vi "Two-TryGuessingGame_Branyon.vi"() -> ()   [LabVIEW 2019]
uses:
  <vilib>/numeric/Random Number (Range) U64.vi
  <vilib>/numeric/sub_Random U32.vi
panel:
  in  "Enter Guess 2":bool
  in  "Guess 2":u64
  out "number":u64
  in  "Guess":u64
  in  "Enter Guess":bool
  out "Message":string
  # "Gavin Branyon\n3/24/2024\nTwo-Try Guessing Game"
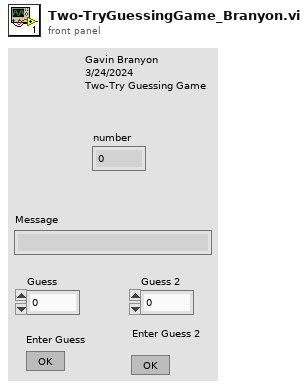
[diagram p1: front panel]
types:
  T1 = enum16{"Generate Number", "Guess", "Check Guess", "Check Guess 2", "Hint", "Correct", "Failure", "Guess 2"}
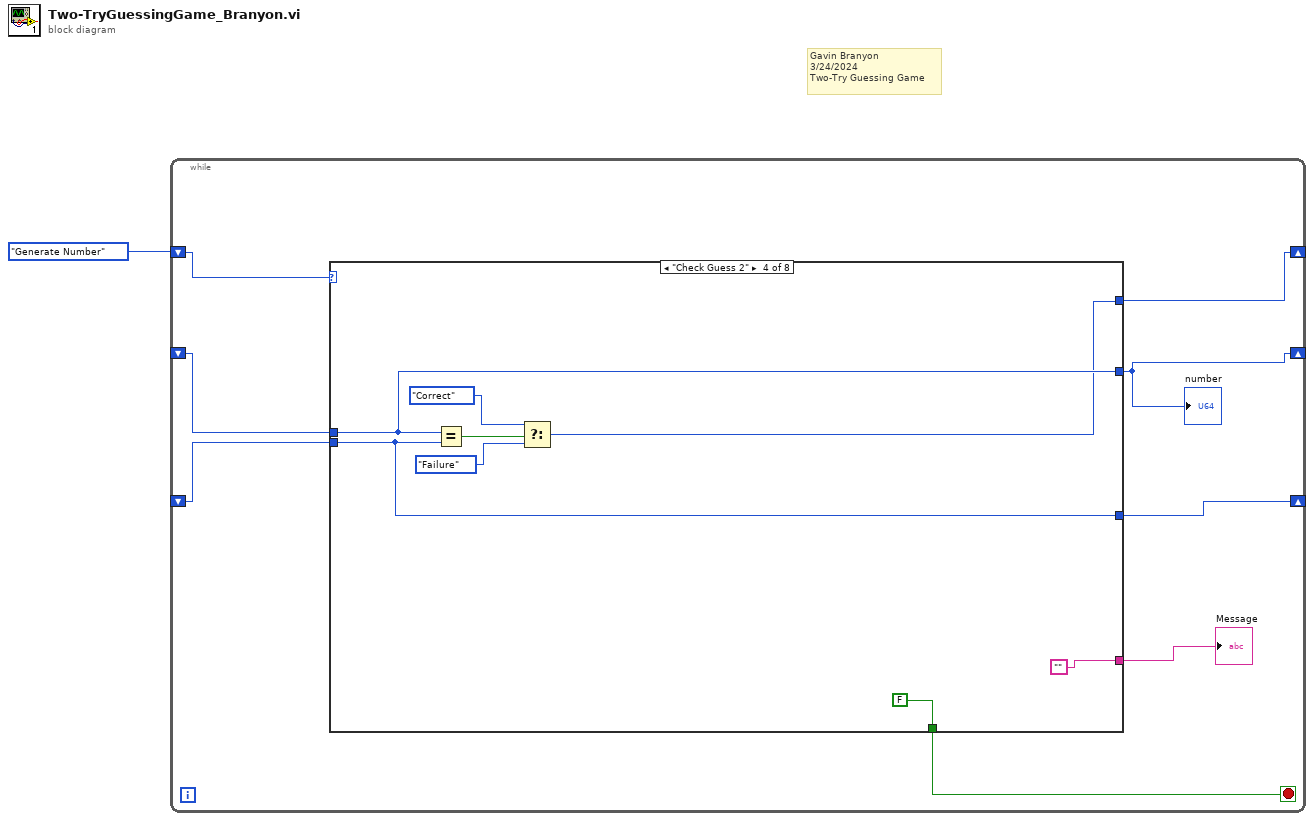
[diagram p0: block diagram]
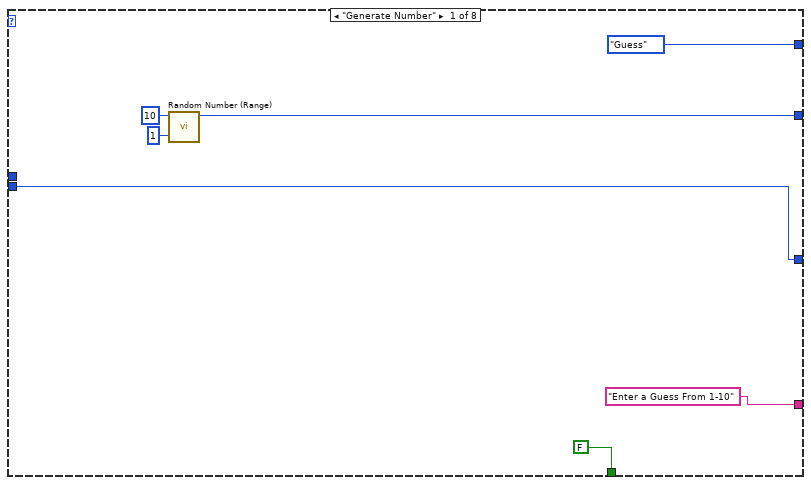
[diagram p2: hidden frame]
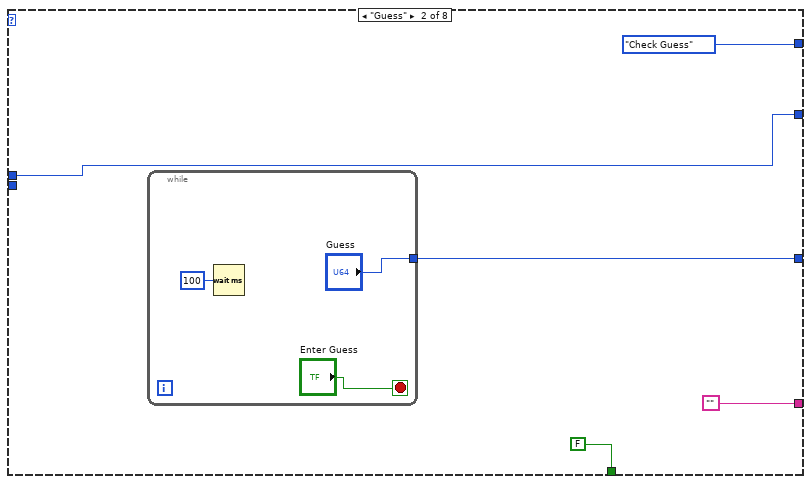
[diagram p3: hidden frame]
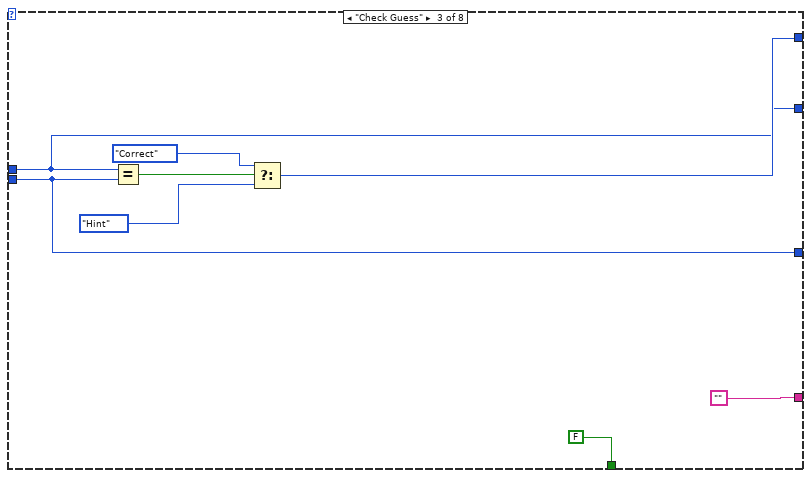
[diagram p4: hidden frame]
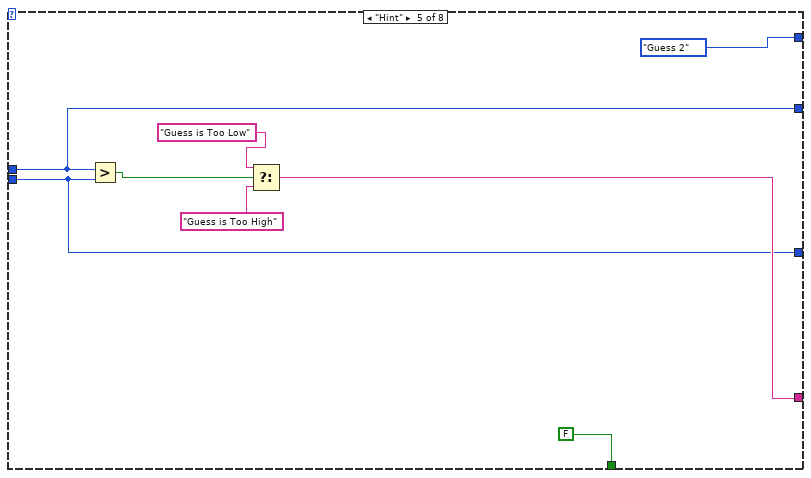
[diagram p5: hidden frame]
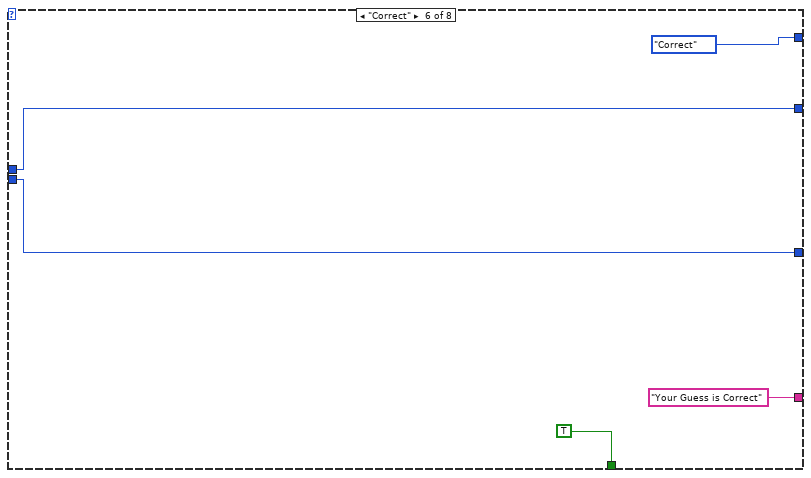
[diagram p6: hidden frame]
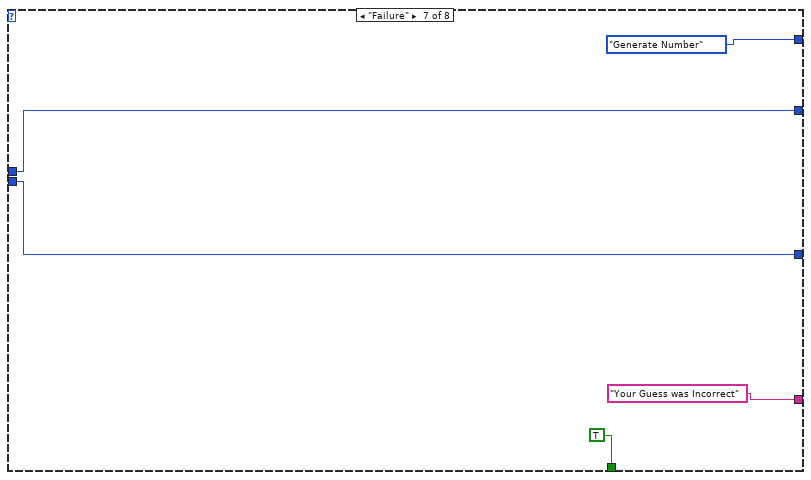
[diagram p7: hidden frame]
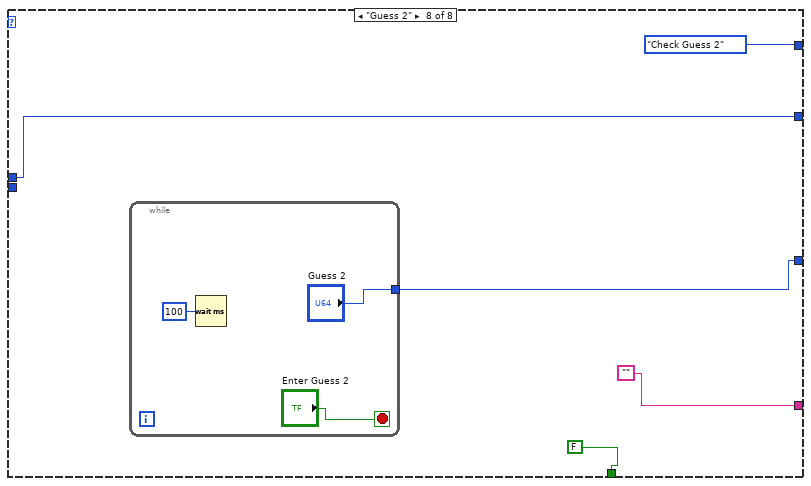
[diagram p8: hidden frame]
diagram:
  # "Gavin Branyon\n3/24/2024\nTwo-Try Guessing Game"
  n1 = while {
    shift-right: [w9] -> _
    shift-left: T1."Generate Number" -> [w3]
    shift-right: [w4] -> _
    shift-left: _ -> [w6]
    shift-right: [w7] -> _
    shift-left: _ -> [w5]
    stop <- w2 stop-if-true
    n2 = case shown="\"Check Guess 2\"" w3 {
      tunnel: [w14 w19 w30 w38 w43 w51 w58 w61] -> w4
      tunnel: [T1."Guess" T1."Check Guess" w31 w37 T1."Guess 2" T1."Correct" T1."Generate Number" T1."Check Guess 2"] -> w9
      tunnel: ["Enter a Guess From 1-10" "" "" "" w45 "Your Guess is Correct" "Your Guess was Incorrect" ""] -> w8
      tunnel: [w12 w21 w29 w39 w44 w52 w57 w62] -> w7
      tunnel: w6 -> [_ w19 w30 w38 w43 w51 w58 w61]
      tunnel: w5 -> [w12 _ w29 w39 w44 w52 w57 _]
      tunnel: [FALSE FALSE FALSE FALSE FALSE TRUE TRUE FALSE] -> w2
      frame "Generate Number" {
        n3 = call-poly <vilib>:"Random Number (Range).vi"("lower bound (0)"=u64 1, "upper bound (100)"=u64 10) -> ("number"=w14:u64)  [unwired: 9 in]
      }
      frame "Guess" {
        n4 = while {
          tunnel: ["Guess"] -> w21
          stop <- "Enter Guess" stop-if-true
          n5 = Wait (ms)(milliseconds to wait=u32 100) -> ()  [unwired: 1 out]
        }
      }
      frame "Check Guess" {
        n6 = Equal?(x=w30, y=w29) -> (x = y?=w32:bool)
        n7 = Select(t=T1."Correct", s=w32, f=T1."Hint") -> (s? t:f=w31:T1)
      }
      frame "Check Guess 2" {
        n8 = Equal?(x=w38, y=w39) -> (x = y?=w40:bool)
        n9 = Select(t=T1."Correct", s=w40, f=T1."Failure") -> (s? t:f=w37:T1)
      }
      frame "Hint" {
        n10 = Greater?(x=w43, y=w44) -> (0:w48:bool)
        n11 = Select(t="Guess is Too Low", s=w48, f="Guess is Too High") -> (s? t:f=w45:string)
      }
      frame "Correct" {
      }
      frame "Failure" {
      }
      frame "Guess 2" {
        n12 = while {
          tunnel: ["Guess 2"] -> w62
          stop <- "Enter Guess 2" stop-if-true
          n13 = Wait (ms)(milliseconds to wait=u32 100) -> ()  [unwired: 1 out]
        }
      }
    }
    "Message" <- w8
    "number" <- w4
  }
